vi "Begin.vi"(7 "error in":errorcluster) -> (0 "error out":errorcluster)   [LabVIEW 2015]
doc: "Called before other user functions, this VI is expected to open initial I/O refnums, load in file data, and do all program initialization. Notice that the <B>error out</B> terminal is simply used for data flow. Wiring it to other structures or subVIs ensures that this VI runs first."
uses:
  <vilib>/Rock Robotics/WPI/DriverStation/WPI_DriverStationRobotMode2.ctl
  <vilib>/Rock Robotics/WPI/Joystick/WPI_JoystickDeviceEnum.ctl
  <vilib>/Rock Robotics/SystemInterfaces/spilib/spi_bus.ctl
  <vilib>/Rock Robotics/SystemInterfaces/DIO/FPGA_DIOPWMChannel.ctl
  <vilib>/Rock Robotics/WPI/SafetyOutput/WPI_SafetyOutputConfigMenu.ctl
  <vilib>/Rock Robotics/SystemInterfaces/DIO/FPGA_DIOChannel.ctl
  <vilib>/Rock Robotics/SystemInterfaces/AI/FPGA_AIChannel.ctl
  <vilib>/Rock Robotics/WPI/Accelerometer/WPI_AccelerometerRange.ctl
  Robot Global Data.vi
  <vilib>/Rock Robotics/WPI/Gyro/WPI_GyroXRS450_SPI_Open.vi
  <vilib>/Rock Robotics/WPI/RobotDrive/WPI_RobotDriveOpen2MotorWithVictorSP.vi
  <vilib>/Rock Robotics/WPI/MotorControl/WPI_MotorControlOpen VictorSP.vi
  <vilib>/Rock Robotics/WPI/Switch/WPI_SwitchOpenLimit.vi
  <vilib>/Rock Robotics/Network Tables/NT Write Boolean.vi
  <vilib>/Rock Robotics/WPI/Accelerometer/InternalAccelerometer/WPI_AccelerometerInternalOpen.vi
  <vilib>/Rock Robotics/WPI/RobotDrive/WPI_RobotDriveOpen4MotorWithVictorSP.vi
  <vilib>/Rock Robotics/WPI/Counter/WPI_CounterDigitalInputToDigitalSource.vi
  <vilib>/Rock Robotics/WPI/Accelerometer/WPI_AccelerometerADXL345 Axes.ctl
  <vilib>/Rock Robotics/WPI/Accelerometer/ADXL362 Range.ctl
  <vilib>/Rock Robotics/WPI/Accelerometer/WPI_AccelerometerADXL362_SPI_Open.vi
  <vilib>/Rock Robotics/WPI/RobotDrive/WPI_RobotDriveOpen2MotorWithTalon.vi
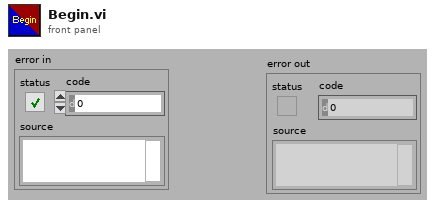
[diagram p1: front panel]
types:
  T1 = typedef "WPI_SafetyOutputConfigMenu.ctl" = enum16{"Enable", "Disable"}
  T2 = typedef "FPGA_DIOPWMChannel.ctl" = enum8{"PWM 0", "PWM 1", "PWM 2", "PWM 3", "PWM 4", "PWM 5", "PWM 6", "PWM 7", "PWM 8", "PWM 9", "PWM MXP 0", "PWM MXP 1", "PWM MXP 2", "PWM MXP 3", "PWM MXP 4", "PWM MXP 5", "PWM MXP 6", "PWM MXP 7", "PWM MXP 8", "PWM MXP 9", "Invalid"}
  T3 = typedef "FPGA_AIChannel.ctl" = enum8{"AI 0", "AI 1", "AI 2", "AI 3", "AI MXP 0", "AI MXP 1", "AI MXP 2", "AI MXP 3", "Invalid"}
  T4 = typedef "WPI_AccelerometerRange.ctl" = enum16{"+/- 2 g", "+/- 4 g", "+/- 8 g"}
  T5 = typedef "FPGA_DIOChannel.ctl" = enum8{"DIO 0", "DIO 1", "DIO 2", "DIO 3", "DIO 4", "DIO 5", "DIO 6", "DIO 7", "DIO 8", "DIO 9", "DIO MXP 0", "DIO MXP 1", "DIO MXP 2", "DIO MXP 3", "DIO MXP 4", "DIO MXP 5", "DIO MXP 6", "DIO MXP 7", "DIO MXP 8", "DIO MXP 9", "DIO MXP 10", "DIO MXP 11", "DIO MXP 12", "DIO MXP 13", "DIO MXP 14", "DIO MXP 15", "Invalid"}
  T6 = typedef "spi_bus.ctl" = enum16{"SPI On-Board, CS0", "SPI On-Board, CS1", "SPI On-Board, CS2", "SPI On-Board, CS3", "SPI MXP", "Invalid"}
  T7 = typedef "WPI_JoystickDeviceEnum.ctl" = enum16{"USB 0", "USB 1", "USB 2", "USB 3", "USB 4", "USB 5"}
  T8 = typedef "WPI_DriverStationRobotMode2.ctl" = enum16{"Autonomous Disabled", "Autonomous Enabled", "Teleop Disabled", "Teleop Enabled", "Disconnected", "Finish", "Test Disabled", "Test Enabled", "Emergency Stopped"}
  T9 = typedef "WPI_RobotDriveDevRef.ctl" = cluster{"DevStatus":errorcluster, "Motors[]":T10[], "Square Inputs":bool, "Max Output":dbl}
  T10 = typedef "WPI_MotorControlDeviceRef.ctl" = cluster{"DeviceStatus":errorcluster, "Type":T11, "PWM":cluster{"PWM Channel":T2, "DeadBand":T12}, "CAN":cluster{"Device Number":u8, "Control Mode":T13, "Semaphore":T14, "Max Vout":dbl, "TalonSRX Control Mode":T15}, "Invert":bool}
  T11 = typedef "WPI_MotorControlType.ctl" = enum16{"PWM", "CAN", "CANTalonSRX"}
  T12 = typedef "WPI_PWMDeadband.ctl" = cluster{"Name":string, "maxPositivePwm":i32, "minPositivePwm":i32, "centerPwm":i32, "maxNegativePwm":i32, "minNegativePwm":i32, "angularRange":u16}
  T13 = typedef "WPI_CANJaguar_ControlMode.ctl" = enum8{"Percent VBus", "Current", "Speed", "Position", "Voltage"}
  T14 = typedef "Semaphore RefNum" = refnum<k1>
  T15 = typedef "WPI_CANTalonSRX_APIControlMode.ctl" = enum8{"Percent VBus", "Speed", "Position", "Slave", "Unchanged / Invalid", "Voltage Compensation", "Current", "Motion Profile"}
  T16 = typedef "WPI_JoystickDevRef.ctl" = cluster{"Device":T7}
  T17 = typedef "WPI_SwitchDevRef.ctl" = cluster{"DevStatus":errorcluster, "DIO Channel":T5, "CntIndex":T18, "Normally Closed":bool}
  T18 = typedef "FPGA_CounterCtrSystemIndex.ctl" = enum8{"Ctr 0", "Ctr 1", "Ctr 2", "Ctr 3", "Ctr 4", "Ctr 5", "Ctr 6", "Ctr 7", "Invalid"}
  T19 = typedef "WPI_PotentiometerDevRef.ctl" = cluster{"DevStatus":errorcluster, "Analog Channel":T3, "Invert Output":bool}
  T20 = typedef "WPI_GyroDevRef.ctl" = cluster{"DevStatus":errorcluster, "Analog Channel":T3, "Offset":dbl, "Gain (VoltsPerDegree/Second)":dbl, "Gyro Type":enum16{"Analog", "XRS450"}, "Handle":i32, "SPI Bus":T6, "Device Found":bool, "Sample Rate":dbl, "Calibrate On Open":bool}
  T21 = typedef "WPI_AccelerometerDevRef.ctl" = cluster{"DevStatus":errorcluster, "Scaling":T22, "Analog Channels":T23, "I2C Bus":T24, "SPI Bus":T6, "Accel Range":T25, "ADXL Axes":T26, "Handle":i32, "Device Address":u8, "Accel Type":enum16{"Analog", "ADXL345 I2C", "ADXL345 SPI", "Internal", "ADXL362 SPI"}}
  T22 = typedef "WPI_AccelerometerScaling.ctl" = cluster{"Gain (VoltsPerG)":dbl, "Center Voltage":dbl}
  T23 = typedef "WPI_AccelerometerAnalogChannels.ctl" = cluster{"X-Axis":T3, "Y-Axis":T3, "Z-Axis":T3}
  T24 = typedef "i2c_bus.ctl" = enum16{"I2C On-Board", "I2C MXP", "Invalid"}
  T25 = typedef "ADXL345 Range.ctl" = u8
  T26 = typedef "WPI_AccelerometerADXL345 Axes.ctl" = cluster{"X-Axis":bool, "Y-Axis":bool, "Z-Axis":bool}
  T27 = typedef "WPI_DigitalInputDevRef.ctl" = cluster{"DevStatus":errorcluster, "DIO Channel":T5}
  T28 = typedef "FPGA_CounterEncoderSourceConvertionLVSourceType.ctl" = cluster{"DevStatus":errorcluster, "AnalogTriggerMode?":bool, "DigitalMode":cluster{"DIO Channel":T29}, "AnalogTriggerMode":cluster{"AnalogTriggerIndex":T30, "OutputType":T31}}
  T29 = typedef "FPGA_DIODigitalSourceChannel.ctl" = enum8{"DIO 0", "DIO 1", "DIO 2", "DIO 3", "DIO 4", "DIO 5", "DIO 6", "DIO 7", "DIO 8", "DIO 9", "DIO MXP 0", "DIO MXP 1", "DIO MXP 2", "DIO MXP 3", "DIO MXP 4", "DIO MXP 5", "DIO MXP 6", "DIO MXP 7", "DIO MXP 8", "DIO MXP 9", "DIO MXP 10", "DIO MXP 11", "DIO MXP 12", "DIO MXP 13", "DIO MXP 14", "DIO MXP 15", "Disabled"}
  T30 = typedef "FPGA_AnalogTriggerIndex.ctl" = enum8{"Trig 0", "Trig 1", "Trig 2", "Trig 3", "Trig 4", "Trig 5", "Trig 6", "Trig 7", "Invalid"}
  T31 = typedef "FPGA_AnalogTriggerOutType.ctl" = enum16{"InWindow", "TriggerState", "Rising", "Falling"}
  T32 = typedef "WPI_EncoderDevRef.ctl" = cluster{"DevStatus":errorcluster, "EncoderIndex":T33, "CounterIndex":T18, "DistancePerCount":dbl, "Decoding Type":T34}
  T33 = typedef "FPGA_EncoderIdx.ctl" = enum8{"Enc 0", "Enc 1", "Enc 2", "Enc 3", "Enc 4", "Enc 5", "Enc 6", "Enc 7", "Invalid"}
  T34 = typedef "WPI_EncoderType.ctl" = enum16{"1x", "2x", "4x"}
  T35 = typedef "ADXL362 Range.ctl" = u8
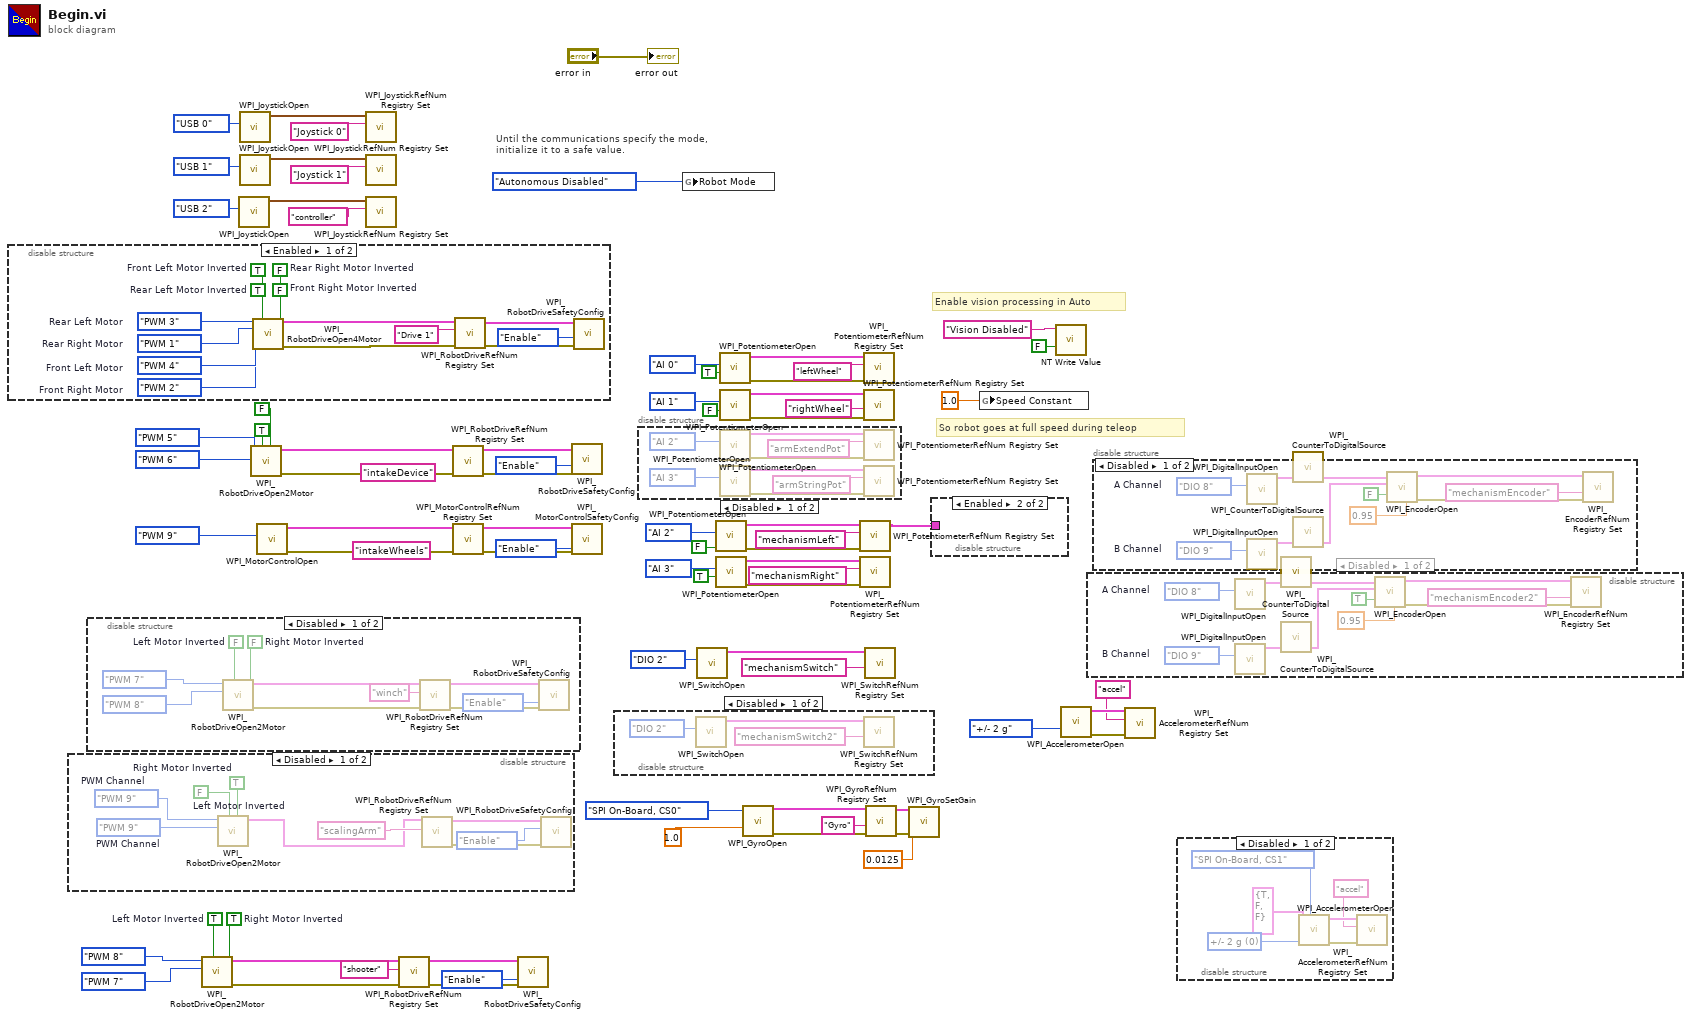
[diagram p0: block diagram]
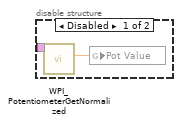
[diagram p2: hidden frame]
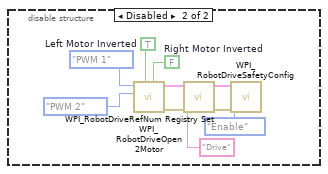
[diagram p9: hidden frame]
diagram:
  w3 = TRUE  # Right Motor Inverted
  w4 = TRUE  # Left Motor Inverted
  # "Enable vision processing in Auto"
  # "So robot goes at full speed during teleop"
  # "Until the communications specify the mode,\ninitialize it to a safe value."
  n1 = disable-structure shown="Enabled" {
    frame Enabled {
      w79 = FALSE  # Rear Right Motor Inverted
      w80 = TRUE  # Rear Left Motor Inverted
      w81 = FALSE  # Front Right Motor Inverted
      w82 = TRUE  # Front Left Motor Inverted
      w83 = FPGA_DIOPWMChannel."PWM 2"  # Front Right Motor
      w84 = FPGA_DIOPWMChannel."PWM 4"  # Front Left Motor
      w87 = FPGA_DIOPWMChannel."PWM 1"  # Rear Right Motor
      w88 = FPGA_DIOPWMChannel."PWM 3"  # Rear Left Motor
      n2 = call-poly <vilib>:"WPI_RobotDriveOpen4Motor.vi"("Rear Left Motor"=w88, "Rear Left Motor Inverted"=w80, "Rear Right Motor Inverted"=w79, "Rear Right Motor"=w87, "Front Left Motor"=w84, "Front Right Motor"=w83, "Front Left Motor Inverted"=w82, "Front Right Motor Inverted"=w81) -> ("RobotDriveDevRef"=w91:T9, "error out"=w89:errorcluster)  [unwired: 6 in]
      n3 = call <vilib>:"WPI_RobotDriveRefNum Registry Set.vi"("error in (no error)"=w89, "refnum name"="Drive 1", "RobotDriveDevRef"=w91) -> ("error out"=w78:errorcluster, "RobotDriveDevRef"=w86:T9)  [unwired: 1 in, 6 out]
      n4 = call <vilib>:"WPI_RobotDriveSafetyConfig.vi"("error in (no error)"=w78, "mode"=WPI_SafetyOutputConfigMenu."Enable", "RobotDriveDevRef"=w86) -> ()  [unwired: 7 in, 2 out]
    }
    frame Disabled {
      w94 = FALSE  # Right Motor Inverted
      w95 = TRUE  # Left Motor Inverted
      n5 = call-poly <vilib>:"WPI_RobotDriveOpen2Motor.vi"("Right Motor Inverted"=w94, "Left Motor Inverted"=w95, "Right Motor"=FPGA_DIOPWMChannel."PWM 2", "Left Motor"=FPGA_DIOPWMChannel."PWM 1") -> ("error out"=w101:errorcluster, "RobotDriveDevRef"=w100:T9)  [unwired: 6 in]
      n6 = call <vilib>:"WPI_RobotDriveRefNum Registry Set.vi"("error in (no error)"=w101, "refnum name"="Drive", "RobotDriveDevRef"=w100) -> ("error out"=w99:errorcluster, "RobotDriveDevRef"=w98:T9)  [unwired: 7 in]
      n7 = call <vilib>:"WPI_RobotDriveSafetyConfig.vi"("error in (no error)"=w99, "mode"=WPI_SafetyOutputConfigMenu."Enable", "RobotDriveDevRef"=w98) -> ()  [unwired: 7 in, 2 out]
    }
  }
  n8 = disable-structure shown="Disabled" {
    frame Disabled {
      w102 = TRUE  # Right Motor Inverted
      w103 = FALSE  # Left Motor Inverted
      w104 = FPGA_DIOPWMChannel."PWM 9"  # PWM Channel
      w110 = FPGA_DIOPWMChannel."PWM 9"  # PWM Channel
      n9 = call-poly <vilib>:"WPI_RobotDriveOpen2Motor.vi"("Right Motor Inverted"=w102, "Left Motor Inverted"=w103, "Right Motor"=w110, "Left Motor"=w104) -> ("RobotDriveDevRef"=w105:T9)  [unwired: 6 in, 1 out]
      n10 = call <vilib>:"WPI_RobotDriveRefNum Registry Set.vi"("refnum name"="scalingArm", "RobotDriveDevRef"=w105) -> ("error out"=w108:errorcluster, "RobotDriveDevRef"=w109:T9)  [unwired: 8 in]
      n11 = call <vilib>:"WPI_RobotDriveSafetyConfig.vi"("error in (no error)"=w108, "mode"=WPI_SafetyOutputConfigMenu."Enable", "RobotDriveDevRef"=w109) -> ()  [unwired: 7 in, 2 out]
    }
    frame Enabled {
    }
  }
  n12 = disable-structure shown="Disabled" {
    frame Disabled {
      w113 = FALSE  # Right Motor Inverted
      w114 = FALSE  # Left Motor Inverted
      n13 = call-poly <vilib>:"WPI_RobotDriveOpen2Motor.vi"("Right Motor Inverted"=w113, "Left Motor Inverted"=w114, "Right Motor"=FPGA_DIOPWMChannel."PWM 8", "Left Motor"=FPGA_DIOPWMChannel."PWM 7") -> ("error out"=w120:errorcluster, "RobotDriveDevRef"=w119:T9)  [unwired: 6 in]
      n14 = call <vilib>:"WPI_RobotDriveRefNum Registry Set.vi"("error in (no error)"=w120, "refnum name"="winch", "RobotDriveDevRef"=w119) -> ("error out"=w118:errorcluster, "RobotDriveDevRef"=w117:T9)  [unwired: 7 in]
      n15 = call <vilib>:"WPI_RobotDriveSafetyConfig.vi"("error in (no error)"=w118, "mode"=WPI_SafetyOutputConfigMenu."Enable", "RobotDriveDevRef"=w117) -> ()  [unwired: 7 in, 2 out]
    }
    frame Enabled {
    }
  }
  n16 = call-poly <vilib>:"WPI_RobotDriveOpen2Motor.vi"("Right Motor Inverted"=w3, "Left Motor Inverted"=w4, "Right Motor"=FPGA_DIOPWMChannel."PWM 7", "Left Motor"=FPGA_DIOPWMChannel."PWM 8") -> ("error out"=w10:errorcluster, "RobotDriveDevRef"=w9:T9)  [unwired: 6 in]
  n17 = call <vilib>:"WPI_JoystickOpen.vi"("JoystickDevice"=WPI_JoystickDeviceEnum."USB 2") -> ("JoystickDevRef"=w65:T16)  [unwired: 10 in]
  n18 = call <vilib>:"WPI_JoystickOpen.vi"("JoystickDevice"=WPI_JoystickDeviceEnum."USB 0") -> ("JoystickDevRef"=w74:T16)  [unwired: 10 in]
  n19 = call <vilib>:"WPI_JoystickOpen.vi"("JoystickDevice"=WPI_JoystickDeviceEnum."USB 1") -> ("JoystickDevRef"=w71:T16)  [unwired: 10 in]
  n20 = call-poly <vilib>:"WPI_RobotDriveOpen2Motor.vi"("Right Motor Inverted"=FALSE, "Left Motor Inverted"=TRUE, "Right Motor"=FPGA_DIOPWMChannel."PWM 6", "Left Motor"=FPGA_DIOPWMChannel."PWM 5") -> ("error out"=w61:errorcluster, "RobotDriveDevRef"=w60:T9)  [unwired: 6 in]
  n21 = call-poly <vilib>:"WPI_MotorControlOpen.vi"("PWM Channel"=FPGA_DIOPWMChannel."PWM 9") -> ("error out"=w49:errorcluster, "MotorControlDeviceRef"=w48:T10)  [unwired: 9 in]
  n22 = call <vilib>:"WPI_JoystickRefNum Registry Set.vi"("refnum name"="Joystick 0", "JoystickDevRef"=w74) -> ()  [unwired: 8 in, 2 out]
  n23 = call <vilib>:"WPI_JoystickRefNum Registry Set.vi"("refnum name"="Joystick 1", "JoystickDevRef"=w71) -> ()  [unwired: 8 in, 2 out]
  n24 = call <vilib>:"WPI_JoystickRefNum Registry Set.vi"("refnum name"="controller", "JoystickDevRef"=w65) -> ()  [unwired: 8 in, 2 out]
  n25 = call <vilib>:"WPI_RobotDriveRefNum Registry Set.vi"("error in (no error)"=w10, "refnum name"="shooter", "RobotDriveDevRef"=w9) -> ("error out"=w8:errorcluster, "RobotDriveDevRef"=w7:T9)  [unwired: 7 in]
  n26 = call <vilib>:"WPI_RobotDriveRefNum Registry Set.vi"("error in (no error)"=w61, "refnum name"="intakeDevice", "RobotDriveDevRef"=w60) -> ("error out"=w59:errorcluster, "RobotDriveDevRef"=w58:T9)  [unwired: 7 in]
  n27 = call <vilib>:"WPI_MotorControlRefNum Registry Set.vi"("error in (no error)"=w49, "refnum name"="intakeWheels", "MotorControlDevRef"=w48) -> ("error out"=w46:errorcluster, "MotorControlDevRef"=w45:T10)  [unwired: 7 in]
  n28 = call <vilib>:"WPI_RobotDriveSafetyConfig.vi"("error in (no error)"=w8, "mode"=WPI_SafetyOutputConfigMenu."Enable", "RobotDriveDevRef"=w7) -> ()  [unwired: 7 in, 2 out]
  n29 = call <vilib>:"WPI_RobotDriveSafetyConfig.vi"("error in (no error)"=w59, "mode"=WPI_SafetyOutputConfigMenu."Enable", "RobotDriveDevRef"=w58) -> ()  [unwired: 7 in, 2 out]
  n30 = call <vilib>:"WPI_MotorControlSafetyConfig.vi"("error in (no error)"=w46, "mode"=WPI_SafetyOutputConfigMenu."Enable", "MotorControlDevRef"=w45) -> ()  [unwired: 7 in, 2 out]
  n31 = disable-structure shown="Disabled" {
    frame Disabled {
      n32 = call-poly <vilib>:"WPI_SwitchOpen.vi"("DIO Channel"=FPGA_DIOChannel."DIO 2") -> ("SwitchDevRef"=w121:T17)  [unwired: 9 in, 1 out]
      n33 = call <vilib>:"WPI_SwitchRefNum Registry Set.vi"("refnum name"="mechanismSwitch2", "SwitchDevRef"=w121) -> ()  [unwired: 8 in, 2 out]
    }
    frame Enabled {
    }
  }
  n34 = disable-structure shown="Disabled" {
    frame Disabled {
      n35 = call <vilib>:"WPI_PotentiometerOpen.vi"("Analog Channel"=FPGA_AIChannel."AI 2") -> ("error out"=w131:errorcluster, "PotDevRef"=w130:T19)  [unwired: 9 in]
      n36 = call <vilib>:"WPI_PotentiometerOpen.vi"("Analog Channel"=FPGA_AIChannel."AI 3") -> ("error out"=w127:errorcluster, "PotDevRef"=w126:T19)  [unwired: 9 in]
      n37 = call <vilib>:"WPI_PotentiometerRefNum Registry Set.vi"("error in (no error)"=w131, "refnum name"="armExtendPot", "PotDevRef"=w130) -> ()  [unwired: 7 in, 2 out]
      n38 = call <vilib>:"WPI_PotentiometerRefNum Registry Set.vi"("error in (no error)"=w127, "refnum name"="armStringPot", "PotDevRef"=w126) -> ()  [unwired: 7 in, 2 out]
    }
    frame Enabled {
    }
  }
  n39 = global write "Robot Global Data.vi" "Robot Mode"(WPI_DriverStationRobotMode2."Autonomous Disabled" ("Robot Mode")) -> ()
  n40 = call-poly <vilib>:"WPI_SwitchOpen.vi"("DIO Channel"=FPGA_DIOChannel."DIO 2") -> ("SwitchDevRef"=w43:T17)  [unwired: 9 in, 1 out]
  n41 = call <vilib>:"WPI_PotentiometerOpen.vi"("Invert Output"=FALSE, "Analog Channel"=FPGA_AIChannel."AI 2") -> ("error out"=w21:errorcluster, "PotDevRef"=w20:T19)  [unwired: 8 in]
  n42 = call <vilib>:"WPI_PotentiometerOpen.vi"("Invert Output"=TRUE, "Analog Channel"=FPGA_AIChannel."AI 3") -> ("error out"=w17:errorcluster, "PotDevRef"=w16:T19)  [unwired: 8 in]
  n43 = call <vilib>:"WPI_PotentiometerOpen.vi"("Invert Output"=TRUE, "Analog Channel"=FPGA_AIChannel."AI 0") -> ("error out"=w40:errorcluster, "PotDevRef"=w39:T19)  [unwired: 8 in]
  n44 = call <vilib>:"WPI_PotentiometerOpen.vi"("Invert Output"=FALSE, "Analog Channel"=FPGA_AIChannel."AI 1") -> ("error out"=w36:errorcluster, "PotDevRef"=w35:T19)  [unwired: 8 in]
  n45 = call-poly <vilib>:"WPI_GyroOpen.vi"("Sample Rate (ms)"=1.0, "SPI Bus"=spi_bus."SPI On-Board, CS0") -> ("error out"=w69:errorcluster, "GyroDevRef"=w68:T20)  [unwired: 8 in]
  n46 = call <vilib>:"WPI_PotentiometerRefNum Registry Set.vi"("error in (no error)"=w21, "refnum name"="mechanismLeft", "PotDevRef"=w20) -> ("PotDevRef"=w11:T19)  [unwired: 7 in, 1 out]
  n47 = call <vilib>:"WPI_PotentiometerRefNum Registry Set.vi"("error in (no error)"=w17, "refnum name"="mechanismRight", "PotDevRef"=w16) -> ()  [unwired: 7 in, 2 out]
  n48 = call <vilib>:"WPI_PotentiometerRefNum Registry Set.vi"("error in (no error)"=w40, "refnum name"="leftWheel", "PotDevRef"=w39) -> ()  [unwired: 7 in, 2 out]
  n49 = call <vilib>:"WPI_PotentiometerRefNum Registry Set.vi"("error in (no error)"=w36, "refnum name"="rightWheel", "PotDevRef"=w35) -> ()  [unwired: 7 in, 2 out]
  n50 = call <vilib>:"WPI_SwitchRefNum Registry Set.vi"("refnum name"="mechanismSwitch", "SwitchDevRef"=w43) -> ()  [unwired: 8 in, 2 out]
  n51 = call <vilib>:"WPI_GyroRefNum Registry Set.vi"("error in (no error)"=w69, "refnum name"="Gyro", "GyroDevRef"=w68) -> ("error out"=w29:errorcluster, "GyroDevRef"=w30:T20)  [unwired: 7 in]
  n52 = call <vilib>:"WPI_GyroSetGain.vi"("error in (no error)"=w29, "Gain (VoltsPerDegree/Second)"=0.0125, "GyroDevRef"=w30) -> ()  [unwired: 7 in, 2 out]
  n53 = disable-structure shown="Enabled" {
    disable-tunnel: w11 -> [w133 _]
    frame Disabled {
      n54 = call <vilib>:"WPI_PotentiometerGetNormalized.vi"("PotDevRef"=w133) -> ("Normalized Value"=w132:dbl)  [unwired: 8 in, 2 out]
      n55 = global write "Robot Global Data.vi" "Pot Value"(w132) -> ()
    }
    frame Enabled {
    }
  }
  n56 = global write "Robot Global Data.vi" "Speed Constant"(1.0 ("Speed Constant")) -> ()
  n57 = call-poly <vilib>:"NT Write Value.vi"("Boolean"=FALSE, "Name"="Vision Disabled") -> ()  [unwired: 9 in, 1 out]
  n58 = call-poly <vilib>:"WPI_AccelerometerOpen.vi"("Accel Range"=WPI_AccelerometerRange."+/- 2 g") -> ("error out"=w22:errorcluster, "AccelerometerDevRef"=w24:T21)  [unwired: 9 in]
  n59 = disable-structure shown="Disabled" {
    frame Disabled {
      w134 = FPGA_DIOChannel."DIO 9"  # B Channel
      w135 = FPGA_DIOChannel."DIO 8"  # A Channel
      n60 = call <vilib>:"WPI_DigitalInputOpen.vi"("DIO Channel"=w135) -> ("DigitalInputDevRef"=w138:T27)  [unwired: 1 in, 9 out]
      n61 = call <vilib>:"WPI_DigitalInputOpen.vi"("DIO Channel"=w134) -> ("DigitalInputDevRef"=w137:T27)  [unwired: 1 in, 9 out]
      n62 = call-poly <vilib>:"WPI_CounterToDigitalSource.vi"("DigitalInputDevRef"=w138) -> ("Digital Source"=w139:T28)  [unwired: 6 out]
      n63 = call-poly <vilib>:"WPI_CounterToDigitalSource.vi"("DigitalInputDevRef"=w137) -> ("Digital Source"=w136:T28)  [unwired: 6 out]
      n64 = call <vilib>:"WPI_EncoderOpen.vi"("DistancePerCount"=0.95, "Invert Direction (False)"=TRUE, "BSource"=w136, "ASource"=w139) -> ("error out"=w140:errorcluster, "EncoderDevRef"=w141:T32)  [unwired: 4 in, 2 out]
      n65 = call <vilib>:"WPI_EncoderRefNum Registry Set.vi"("error in (no error)"=w140, "refnum name"="mechanismEncoder2", "EncoderDevRef"=w141) -> ()  [unwired: 7 in, 2 out]
    }
    frame Enabled {
    }
  }
  n66 = disable-structure shown="Disabled" {
    frame Disabled {
      w155 = FPGA_DIOChannel."DIO 9"  # B Channel
      w154 = FPGA_DIOChannel."DIO 8"  # A Channel
      n67 = call <vilib>:"WPI_DigitalInputOpen.vi"("DIO Channel"=w154) -> ("DigitalInputDevRef"=w151:T27)  [unwired: 1 in, 9 out]
      n68 = call <vilib>:"WPI_DigitalInputOpen.vi"("DIO Channel"=w155) -> ("DigitalInputDevRef"=w152:T27)  [unwired: 1 in, 9 out]
      n69 = call-poly <vilib>:"WPI_CounterToDigitalSource.vi"("DigitalInputDevRef"=w151) -> ("Digital Source"=w150:T28)  [unwired: 6 out]
      n70 = call-poly <vilib>:"WPI_CounterToDigitalSource.vi"("DigitalInputDevRef"=w152) -> ("Digital Source"=w153:T28)  [unwired: 6 out]
      n71 = call <vilib>:"WPI_EncoderOpen.vi"("DistancePerCount"=0.95, "Invert Direction (False)"=FALSE, "BSource"=w153, "ASource"=w150) -> ("error out"=w149:errorcluster, "EncoderDevRef"=w148:T32)  [unwired: 4 in, 2 out]
      n72 = call <vilib>:"WPI_EncoderRefNum Registry Set.vi"("error in (no error)"=w149, "refnum name"="mechanismEncoder", "EncoderDevRef"=w148) -> ()  [unwired: 7 in, 2 out]
    }
    frame Enabled {
    }
  }
  n73 = call <vilib>:"WPI_AccelerometerRefNum Registry Set.vi"("error in (no error)"=w22, "refnum name"="accel", "AccelerometerDevRef"=w24) -> ()  [unwired: 7 in, 2 out]
  n74 = disable-structure shown="Disabled" {
    frame Disabled {
      w156 = T35 0 items=["+/- 2 g", "+/- 4 g", "+/- 8 g"] ("Accel Range")
      n75 = call-poly <vilib>:"WPI_AccelerometerOpen.vi"("SPI Bus"=spi_bus."SPI On-Board, CS1", "Accel Range"=w156, "ADXL345 Axes"=T26 {"X-Axis"=TRUE, "Y-Axis"=FALSE, "Z-Axis"=FALSE}) -> ("error out"=w161:errorcluster, "AccelerometerDevRef"=w160:T21)  [unwired: 7 in]
      n76 = call <vilib>:"WPI_AccelerometerRefNum Registry Set.vi"("error in (no error)"=w161, "refnum name"="accel", "AccelerometerDevRef"=w160) -> ()  [unwired: 7 in, 2 out]
    }
    frame Enabled {
    }
  }
  "error out" <- "error in"
